vi "LIA Debugging FPGA.vi"() -> ()   [LabVIEW 2017]
uses:
  <instrlib>/_niInstr/Streaming/v1/Common/Stream State.ctl
  <instrlib>/_niInstr/Data Trigger/v1/Shared/Public/Edge Configuration FXP(+-,18,1).ctl
  <instrlib>/_niInstr/Data Trigger/v1/Shared/Public/Edge Configuration Trigger Slope.ctl
  <vilib>/Platform/TimedLoop/XDataNode/timing_clust.ctl
  <vilib>/Platform/TimedLoop/XDataNode/nitl_modes.ctl
  <vilib>/Platform/TimedLoop/XDataNode/wakeup.ctl
  <instrlib>/_niInstr/DSP/v1/Shared/Public/IQ Data.ctl
  <vilib>/rvi/Emulation/niFpgaSctlEmulationGetInTimedLoop.vi
  <vilib>/rvi/Emulation/niFpgaEmulationReportErrorSimple.vi
  <vilib>/rvi/Emulation/niFpgaGetClockAttributes.vi
  <vilib>/rvi/Emulation/niFpgaCriticalErrorInLSC.vi
  <instrlib>/_niInstr/DSP/v1/FPGA/Public/Sub VIs/Frequency Shift/Frequency Shift - 1 spc.vi
  <instrlib>/_niInstr/DSP/v1/FPGA/Public/Sub VIs/Fractional Decimator/Fractional Decimator - 1 spc - 2x oc.vi
  <instrlib>/_niInstr/DSP/v1/FPGA/Public/Sub VIs/Fractional Decimator/Fractional Decimator - 10 cps - 1x oc.vi
  <userlib>/_NI Noise Generation IP/FPGA/Public/Low Level/AWGN FXP23x2.vi
  <instrlib>/_niInstr/DSP/v1/FPGA/Public/Sub VIs/Frequency Shift/Frequency Shift - 2 spc.vi
  <vilib>/rvi/eio/common/nirviEmuTemplateMethod_errors.vi
  <vilib>/Platform/TimedLoop/XDataNode/XDataNode.xnode
  <instrlib>/_niInstr/DSP/v1/Xnodes/Public/Frequency Shift/niInstr DSP v1 Frequency Shift FPGA.xnode
  <vilib>/rvi/FXPMathLib/FxpMul/XNode/nifxpmath_Multiplier.xnode
  <vilib>/rvi/FXPMathLib/FxpAdd/XNode/nifxpmath_Add.xnode
  <vilib>/eio/EIONode/EIONode.xnode
  <vilib>/Platform/TimedLoop/XDataNode/XDNodeRunTimeDep.lvlib
  <instrlib>/_niInstr/Basic Elements/v1/FPGA/niInstr Basic Elements v1 FPGA.lvlib
  <instrlib>/_niInstr/DSP/v1/Shared/niInstr DSP v1 Shared.lvlib
  <instrlib>/_niInstr/DSP/v1/FPGA/niInstr DSP v1 FPGA.lvlib
  Program Files (x86)/National Instruments/LabVIEW 2017/examples/Lock-In Amplifier/_NI PLL IP/FPGA/NI PLL IP FPGA.lvlib
  Program Files (x86)/National Instruments/LabVIEW 2017/examples/Lock-In Amplifier/lib/fpga/Lock-In Amplifier Example FPGA.lvlib
  <instrlib>/_niInstr/Streaming/v1/Common/niInstr Streaming v1 Common.lvlib
  <userlib>/_NI Noise Generation IP/FPGA/NI Noise Generation IP FPGA v2.lvlib
  <vilib>/rvi/FXPMathLib/sim/FxpSim.dll
  <instrlib>/_niInstr/Data Trigger/v1/Shared/niInstr Data Trigger v1 Shared.lvlib
panel:
  in  "lock-in.decimator 1":enum16{"None", "FIR"}(ring)
  in  "lock-in.fir2 fs":fxp<+,48,1>
  in  "nco.enable 0":bool=TRUE
  in  "nco.reset 0":bool
  in  "nco.frequency 0":fxp<+/-,48,0>
  in  "lock-in.fir fs":fxp<+,48,1>
  in  "lock-in.decimator 0":enum16{"None", "CIC", "FIR", "4HB"}(ring)
  in  "dpll.reset 1":bool
  in  "dpll.enable 1":bool
  in  "dpll.q 1":fxp<+/-,48,0>
  in  "dpll.m 1":i8
  in  "dpll.config 1":T1
  out "dpll.vco output 1":fxp<+/-,48,0>
  in  "dpll.channel 1":i32
  in  "dpll.channel 0":i32
  out "dpll.vco output 0":fxp<+/-,48,0>
  in  "dpll.config 0":T1
  in  "dpll.m 0":i8
  in  "dpll.q 0":fxp<+/-,48,0>
  in  "dpll.enable 0":bool
  in  "dpll.reset 0":bool
  in  "lock-in.enable 3":bool
  in  "lock-in.enable 2":bool
  in  "lock-in.enable 1":bool
  in  "lock-in.carrier 3":fxp<+/-,48,0>
  in  "lock-in.carrier 2":fxp<+/-,48,0>
  in  "lock-in.enable 0":bool
  in  "lock-in.channel select 3":i32
  in  "lock-in.carrier select 3":i32
  in  "lock-in.cic config valid 3":bool
  in  "lock-in.cic config 3":cluster{"factor":fxp<+,16,16>, "shift":i16}
  in  "lock-in.reset 3":bool
  out "stream.state 3":T3 caption="stream.state 0"
  out "stream.samples transferred 3":u64 caption="stream.samples transferred 0"
  out "stream.metadata 3":u64 caption="stream.metadata 0"
  in  "stream.num samples 3":u64 caption="stream.num samples 0"
  in  "stream.request state 3":T3 caption="stream.request state 0"
  in  "lock-in.channel select 2":i32
  in  "lock-in.carrier select 2":i32
  in  "lock-in.cic config valid 2":bool
  in  "lock-in.cic config 2":cluster{"factor":fxp<+,16,16>, "shift":i16}
  in  "lock-in.reset 2":bool
  out "stream.state 2":T3 caption="stream.state 0"
  out "stream.samples transferred 2":u64 caption="stream.samples transferred 0"
  out "stream.metadata 2":u64 caption="stream.metadata 0"
  in  "stream.num samples 2":u64 caption="stream.num samples 0"
  in  "stream.request state 2":T3 caption="stream.request state 0"
  out "pll.vco output 0":fxp<+/-,48,0>
  out "pll.vco output 1":fxp<+/-,48,0>
  out "stream.metadata 4":u64 caption="stream.metadata 0"
  out "stream.samples transferred 4":u64 caption="stream.samples transferred 0"
  out "stream.state 4":T3 caption="stream.state 0"
  in  "stream.request state 4":T3 caption="stream.request state 0"
  in  "stream.num samples 4":u64 caption="stream.num samples 0"
  in  "preview.channel select":i32
  in  "ao.reset 3":bool
  in  "ao.carrier 2":fxp<+/-,48,0>=0.010000000000001563
  in  "ao.level 2":fxp<+/-,18,1>
  in  "ao.reset 2":bool
  in  "ao.carrier 1":fxp<+/-,48,0>=0.010000000000001563
  in  "ao.level 1":fxp<+/-,18,1>
  in  "ao.reset 1":bool
  in  "ao.reset 0":bool
  in  "ao.carrier 0":fxp<+/-,48,0>=0.010000000000001563
  in  "ao.level 0":fxp<+/-,18,1>
  in  "lock-in.channel select 1":i32
  in  "lock-in.channel select 0":i32
  in  "stream.request state 1":T3 caption="stream.request state 0"
  in  "stream.num samples 1":u64 caption="stream.num samples 0"
  out "stream.metadata 1":u64 caption="stream.metadata 0"
  out "stream.samples transferred 1":u64 caption="stream.samples transferred 0"
  out "stream.state 1":T3 caption="stream.state 0"
  in  "lock-in.reset 1":bool
  in  "lock-in.cic config 1":cluster{"factor":fxp<+,16,16>, "shift":i16}
  in  "lock-in.cic config valid 1":bool
  in  "lock-in.carrier select 1":i32
  in  "lock-in.carrier select 0":i32
  in  "lock-in.cic config valid 0":bool
  in  "lock-in.cic config 0":cluster{"factor":fxp<+,16,16>, "shift":i16}
  in  "lock-in.reset 0":bool
  in  "lock-in.carrier 1":fxp<+/-,48,0>
  in  "lock-in.carrier 0":fxp<+/-,48,0>
  in  "ao.level 3":fxp<+/-,18,1>
  in  "pll.channel 1":i32
  in  "pll.reset 1":bool
  in  "pll.enable 1":bool
  in  "pll.config 1":T4={"quiescent frequency"=0.10000000000000142, "compensation"=0.0, "psd gain"=-18, "loop filter"={"order"=4, "cutoff"=6}}
  in  "pll.channel 0":i32
  in  "ao.noise gain 3":fxp<+,18,1>=0.01000213623046875
  in  "ao.carrier 3":fxp<+/-,48,0>=0.010000000000001563
  in  "ao.noise seeds 3":fxp<+,23,23>[](array[numeric])=[1.0, 12323.0]
  in  "pll.reset 0":bool
  in  "pll.enable 0":bool
  in  "stream.request state 0":T3
  in  "stream.num samples 0":u64
  out "stream.metadata 0":u64
  out "stream.samples transferred 0":u64
  out "stream.state 0":T3
  in  "pll.config 0":T4={"quiescent frequency"=0.10000000000000142, "compensation"=0.0, "psd gain"=-18, "loop filter"={"order"=4, "cutoff"=6}}
  out "IO Module\\InitDone":bool
  out "IO Module\\User Error":u32
  in  "IO Module\\User Command":u32
  in  "IO Module\\User Command Valid":bool
  out "IO Module\\User Command Ready":bool
  in  "IO Module\\User Command Arg 0":u32
  in  "IO Module\\User Command Arg 1":u32
  out "IO Module\\User Command Error":u16
  out "IO Module\\User Command Return":u32
  out "IO Module\\User Command Return Valid":bool
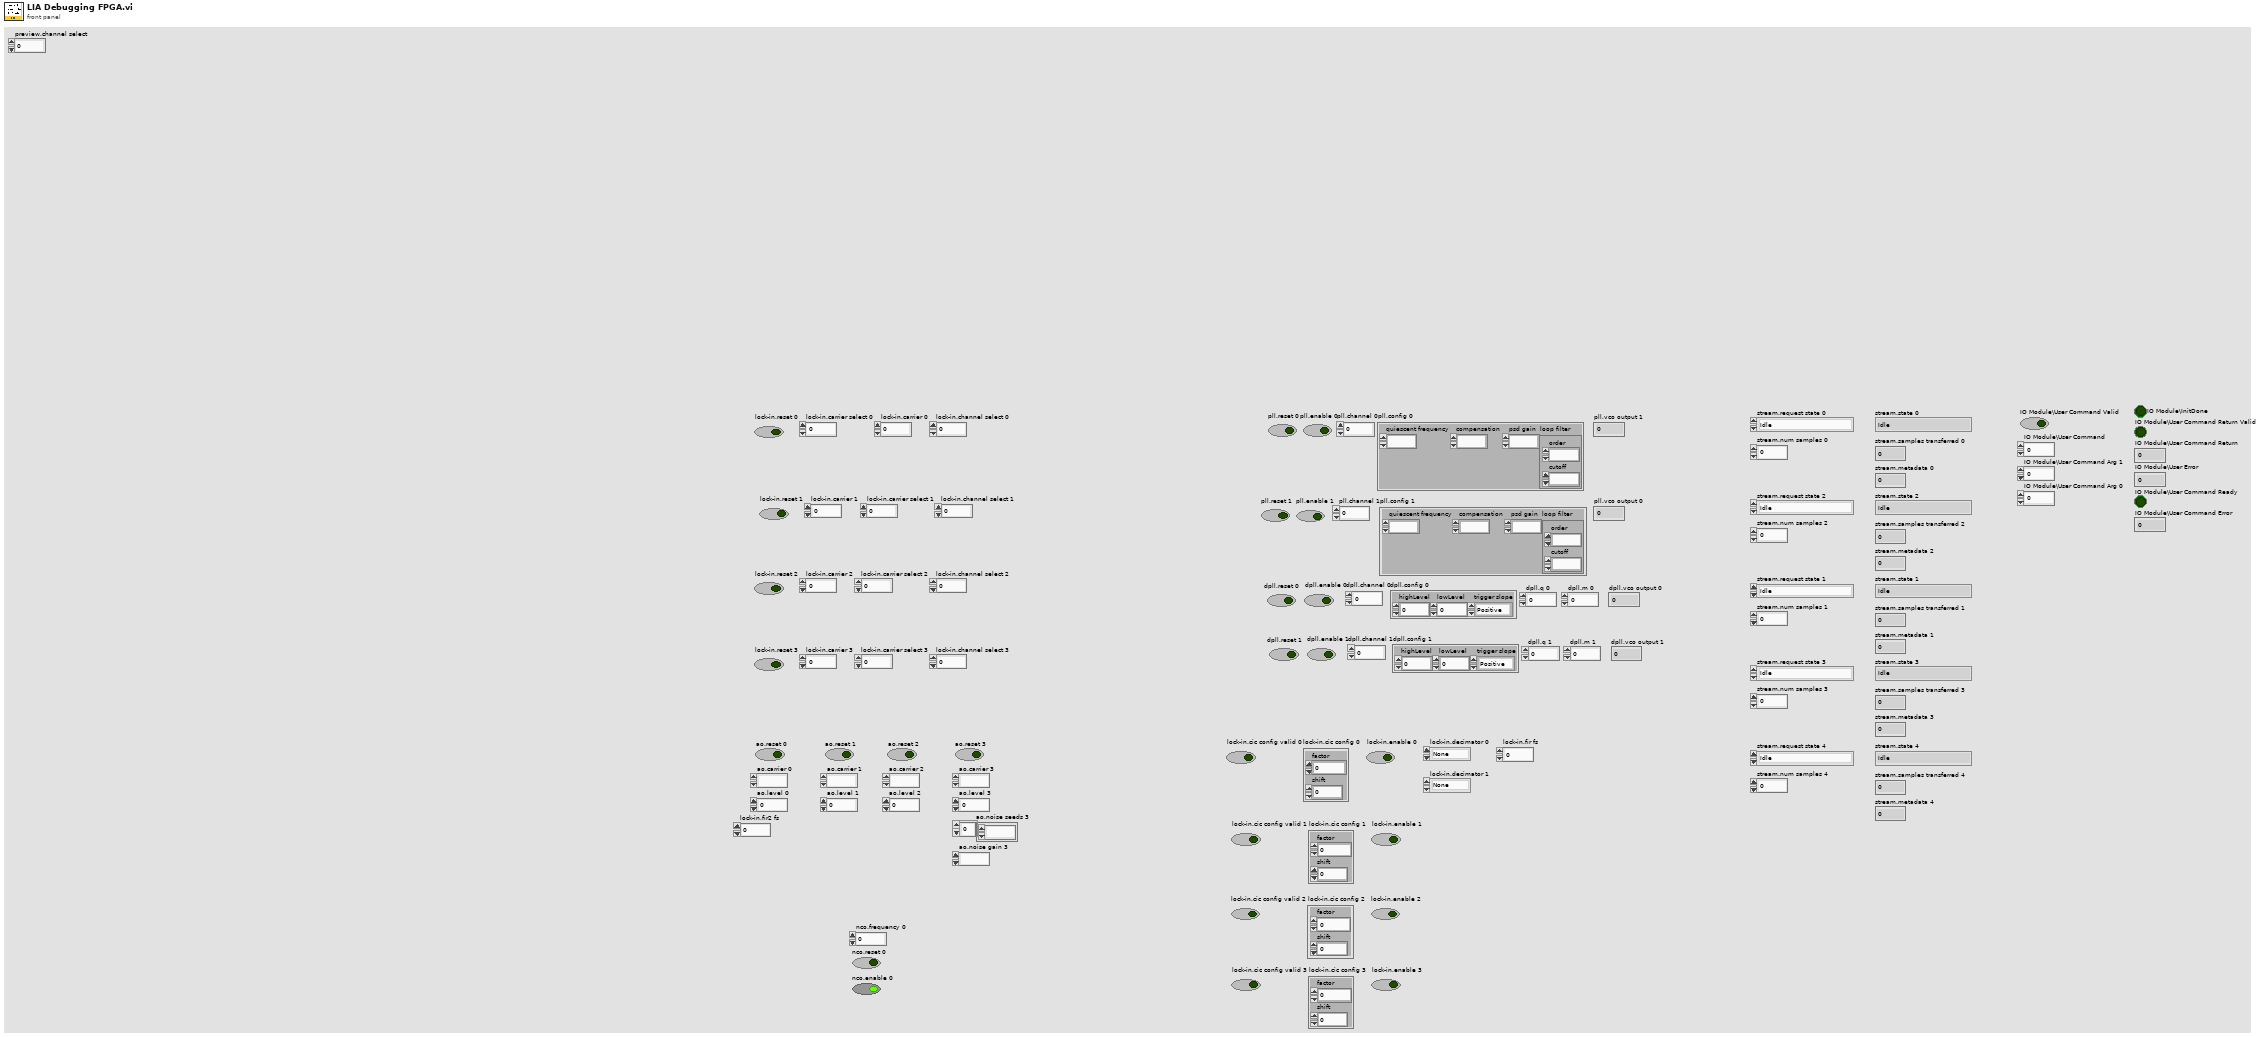
[diagram p1: front panel]
types:
  T1 = typedef "niInstr Data Trigger v1 Shared.lvlib/Edge Configuration FXP(+-,18,1).ctl" = cluster{"highLevel":fxp<+/-,18,1>, "lowLevel":fxp<+/-,18,1>, "trigger slope":T2}
  T2 = typedef "niInstr Data Trigger v1 Shared.lvlib/Edge Configuration Trigger Slope.ctl" = enum8{"Positive", "Negative"}
  T3 = typedef "niInstr Streaming v1 Common.lvlib/Stream State.ctl" = enum8{"Idle", "Finite Transfer", "Continuous", "Done", "Error", "Not Ready", "Cancel"}
  T4 = cluster{"quiescent frequency":fxp<+/-,48,0>, "compensation":fxp<+/-,18,3>, "psd gain":i16, "loop filter":cluster{"order":i32, "cutoff":i8}}
  T5 = typedef "XDNodeRunTimeDep.lvlib/timing_clust.ctl" = cluster{"Expected End [f-1]":u64, "Actual End [f-1]":u64, "Finished Late? [f-1]":bool, "Expected End [i-1]":u64, "Actual End [i-1]":u64, "Finished Late? [i-1]":bool, "Expected Start [i]":u64, "Actual Start [i]":u64, "Expected Start [f]":u64, "Actual Start [f]":u64, "Source Name":string, "Structure Name":string, "Period":i64, "Deadline":i64, "Offset":i64, "Start":i64, "Priority":i32, "Timeout":i32, "Mode":T6, "Wakeup Reason":T7, "Error":errorcluster, "Source Type":string, "Secondary Source Type":string, "Global End Time":u64, "Global Start Time":u64, "Frame Duration":u64, "Iteration Duration":u64, "Assigned CPU":i32, "I/O Scan Engine Mode":u32}
  T6 = typedef "XDNodeRunTimeDep.lvlib/nitl_modes.ctl" = enum32{"No Change", "Process missed periods, maintain original phase", "Discard missed periods, maintain original phase", "Process missed periods, ignore original phase", "Discard missed periods, ignore original phase"}
  T7 = typedef "XDNodeRunTimeDep.lvlib/wakeup.ctl" = enum32{"Normal", "Aborted", "Asynchronous wakeup", "Timing source error", "Timed loop error", "Timeout"}
  T8 = cluster{"stream.num samples 0":u64, "stream.request state 0":T3, "stream.index 0":i16}
  T9 = typedef "niInstr DSP v1 Shared.lvlib/IQ Data.ctl" = cluster{"I":fxp<+/-,18,1>, "Q":fxp<+/-,18,1>, "overflow":bool}
  T10 = cluster{"stream.metadata 0":u64, "stream.samples transferred 0":u64, "stream.state 0":T3}
  T11 = typedef "niInstr DSP v1 Shared.lvlib/IQ Data - 25 bit.ctl" = cluster{"I":fxp<+/-,25,1>, "Q":fxp<+/-,25,1>, "overflow":bool}
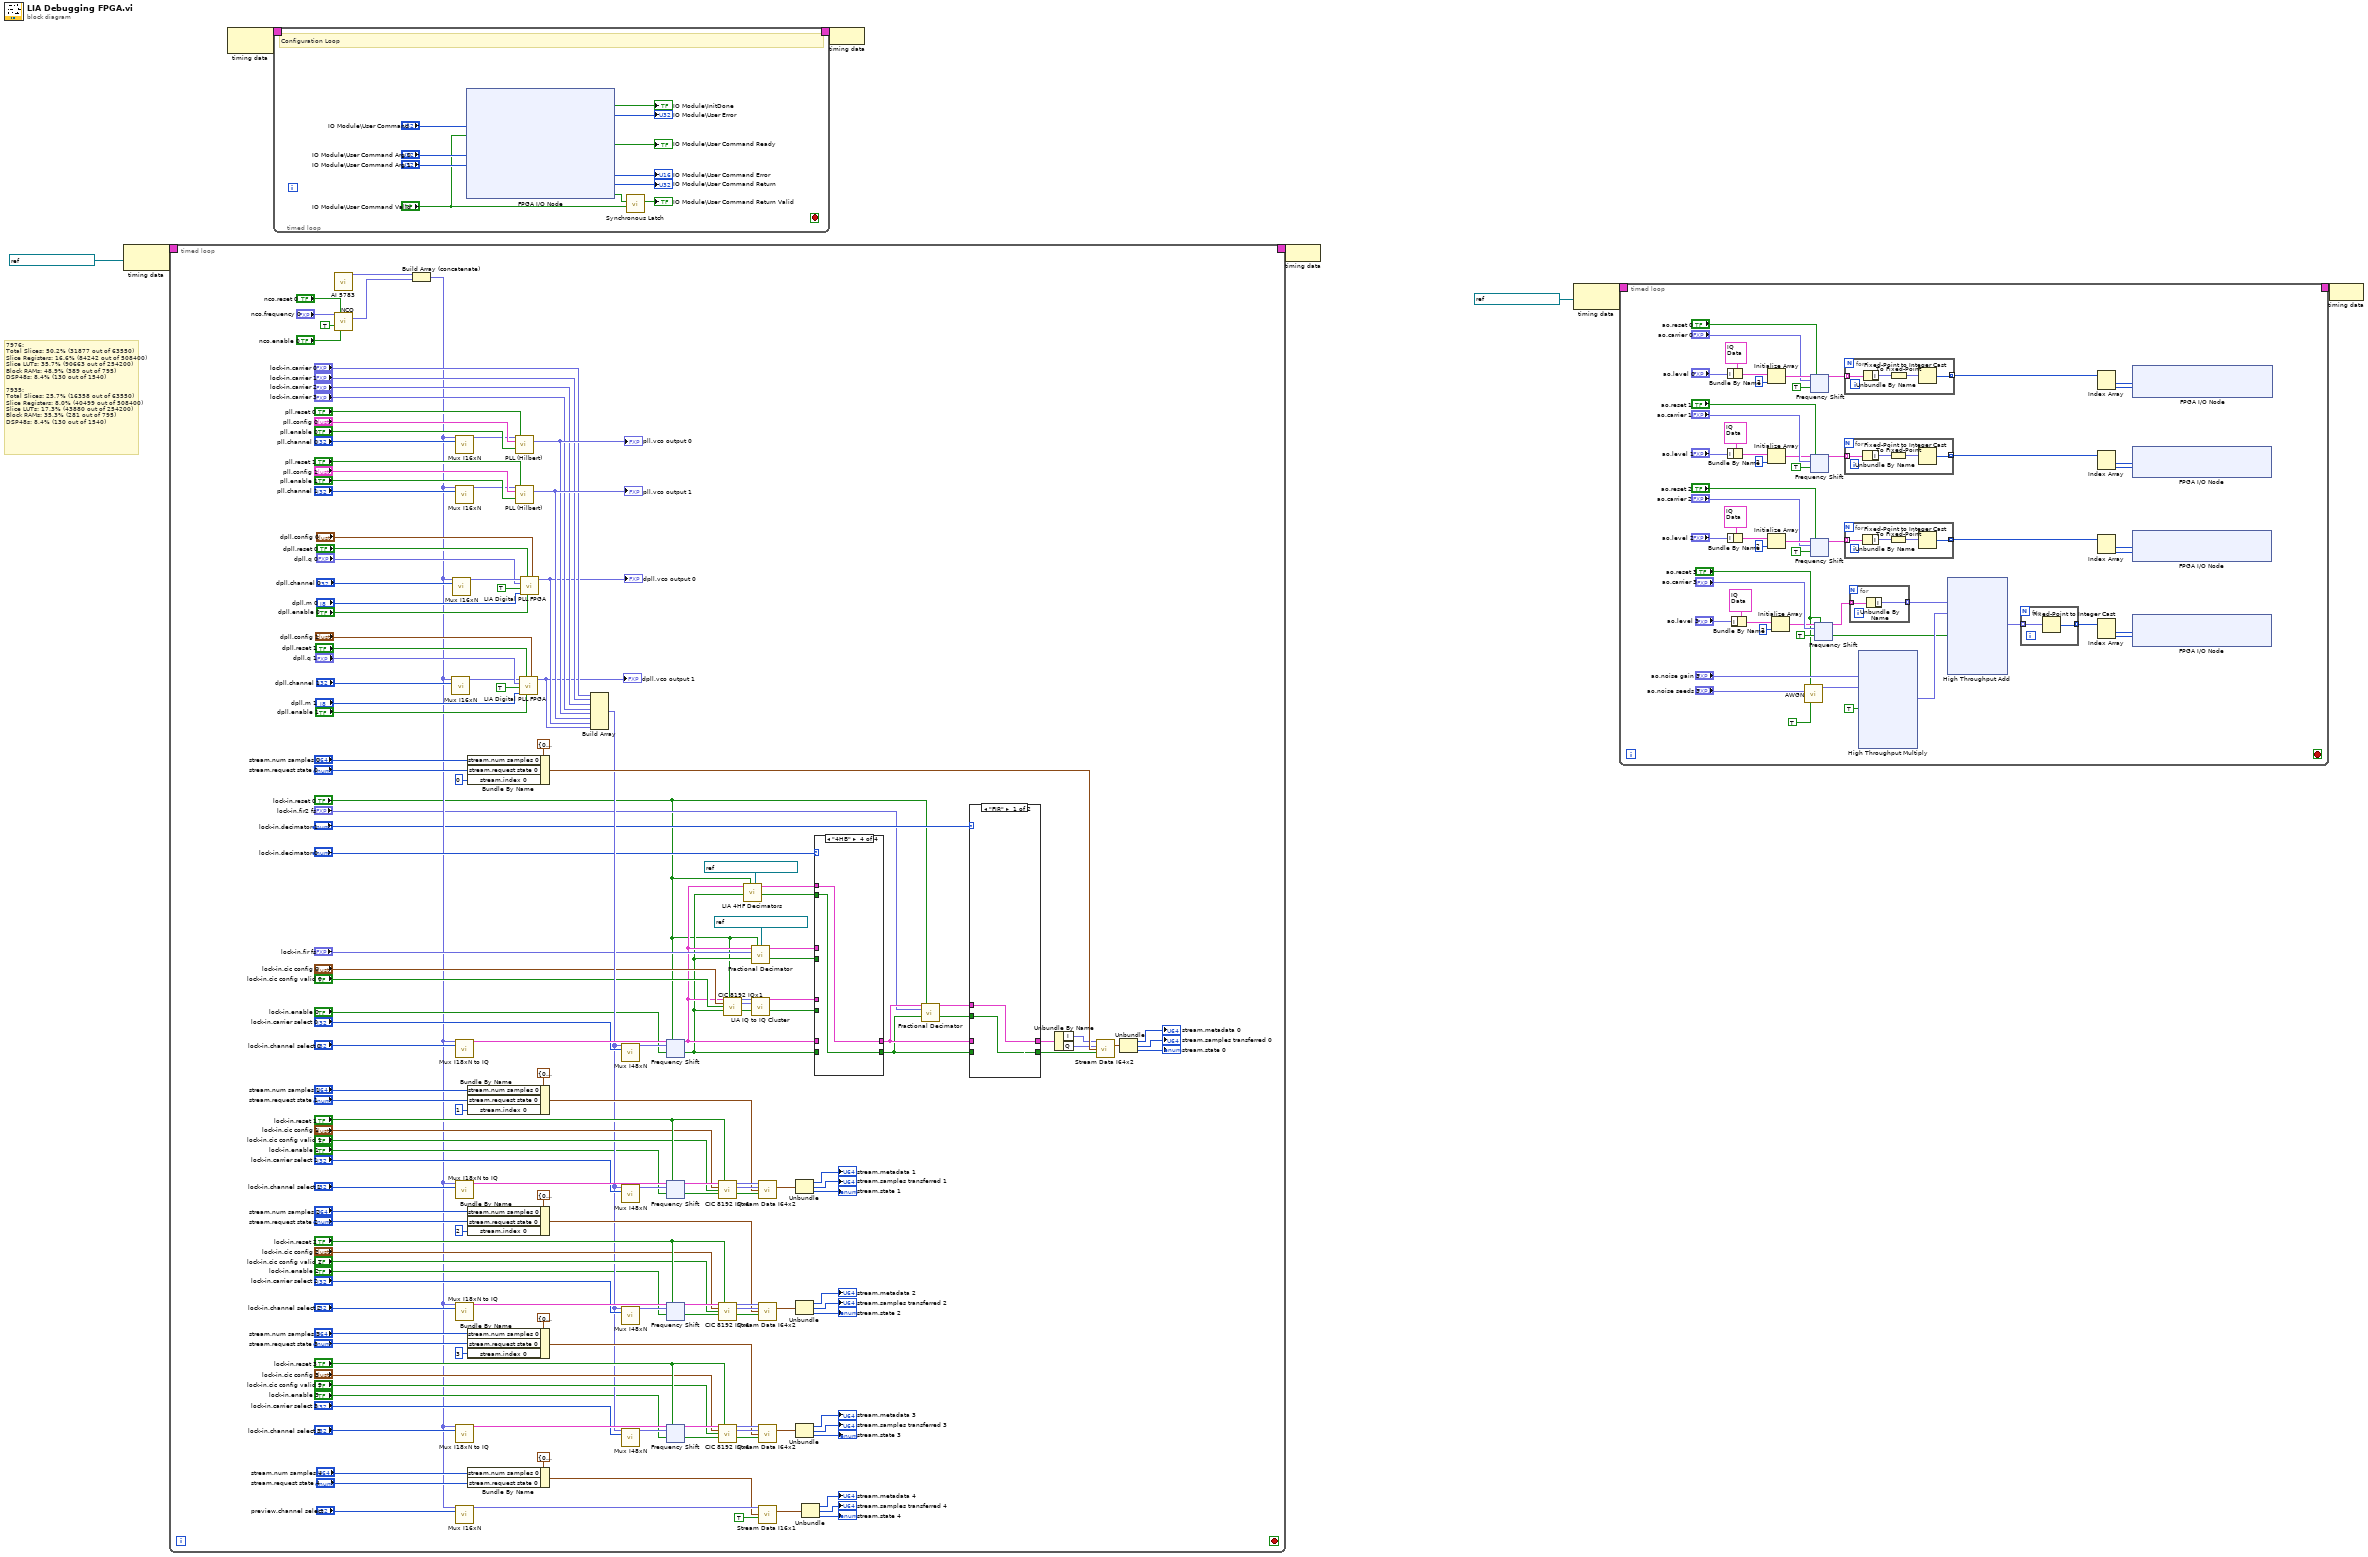
[diagram p0: block diagram]
diagram:
  # "7976:\nTotal Slices: 50.2% (31877 out of 63550)\nSlice Registers: 16.6% (84242 out of 508400)\nSlice LUTs: 35.7% (90663 out of 254200)\nBlock RAMs: 48.9% (389 out of 795)\nDSP48s: 8.4% (130 out of 1540)\n\n7935:\nTotal Slices: 25.7% (16358 out of 63550)\nSlice Registers: 8.0% (40499 out of 508400)\nSlice LUTs: 17.3% (43880 out of 254200)\nBlock RAMs: 35.3% (281 out of 795)\nDSP48s: 8.4% (130 out of 1540)"
  n1 = node-c288(refnum<k21> "IO Module\\Data Clock" ("Source Name")) -> (w8:T5)
  n2 = timed-loop {
    timing: w8 -> [_]
    timing-out: [_] -> w7
    stop <- _ stop-if-true
    n3 = call "AI 5783.vi"() -> ("i18x1"=w43:fxp<+/-,18,1>[])  [unwired: 14 in, 1 out]
    n4 = call <instrlib>:"NCO.vi"("frequency"="nco.frequency 0", "reset"="nco.reset 0", "input valid"=TRUE, "enable (T)"="nco.enable 0") -> ("sine out"=w35:fxp<+/-,18,1>)  [unwired: 9 in, 2 out]
    n5 = Build Array (concatenate)(w43, w35) -> (w36:fxp<+/-,18,1>[])
    n6 = call "Mux I16xN.vi"("i16xn in"=w36, "index"="dpll.channel 1") -> ("i16 out"=w46:fxp<+/-,18,1>)  [unwired: 12 in, 1 out]
    n7 = call "Mux I16xN.vi"("i16xn in"=w36, "index"="dpll.channel 0") -> ("i16 out"=w58:fxp<+/-,18,1>)  [unwired: 12 in, 1 out]
    n8 = call "Mux I16xN.vi"("i16xn in"=w36, "index"="pll.channel 0") -> ("i16 out"=w165:fxp<+/-,18,1>)  [unwired: 12 in, 1 out]
    n9 = call "Mux I16xN.vi"("i16xn in"=w36, "index"="pll.channel 1") -> ("i16 out"=w159:fxp<+/-,18,1>)  [unwired: 12 in, 1 out]
    n10 = call "Mux I18xN to IQ.vi"("i16xn in"=w36, "index"="lock-in.channel select 0") -> ("output"=w158:T9)  [unwired: 12 in, 1 out]
    n11 = call "Mux I18xN to IQ.vi"("i16xn in"=w36, "index"="lock-in.channel select 1") -> ("output"=w145:T9)  [unwired: 12 in, 1 out]
    n12 = call "Mux I18xN to IQ.vi"("i16xn in"=w36, "index"="lock-in.channel select 2") -> ("output"=w111:T9)  [unwired: 12 in, 1 out]
    n13 = call "Mux I18xN to IQ.vi"("i16xn in"=w36, "index"="lock-in.channel select 3") -> ("output"=w90:T9)  [unwired: 12 in, 1 out]
    n14 = call "Mux I16xN.vi"("i16xn in"=w36, "index"="preview.channel select") -> ("i16 out"=w119:fxp<+/-,18,1>)  [unwired: 12 in, 1 out]
    n15 = Bundle By Name(cluster=T8 {"stream.num samples 0"=0, "stream.request state 0"=enum."Idle", "stream.index 0"=0} ("config"), "stream.num samples 0"="stream.num samples 0", "stream.request state 0"="stream.request state 0", "stream.index 0"=i16 0) -> (w148:T8)
    n16 = Bundle By Name(cluster=T8 {"stream.num samples 0"=0, "stream.request state 0"=enum."Idle", "stream.index 0"=0} ("config"), "stream.num samples 0"="stream.num samples 1", "stream.request state 0"="stream.request state 1", "stream.index 0"=i16 1) -> (w127:T8)
    n17 = Bundle By Name(cluster=T8 {"stream.num samples 0"=0, "stream.request state 0"=enum."Idle", "stream.index 0"=0} ("config"), "stream.num samples 0"="stream.num samples 2", "stream.request state 0"="stream.request state 2", "stream.index 0"=i16 2) -> (w93:T8)
    n18 = Bundle By Name(cluster=T8 {"stream.num samples 0"=0, "stream.request state 0"=enum."Idle", "stream.index 0"=0} ("config"), "stream.num samples 0"="stream.num samples 3", "stream.request state 0"="stream.request state 3", "stream.index 0"=i16 3) -> (w72:T8)
    n19 = Bundle By Name(cluster=T8 {"stream.num samples 0"=0, "stream.request state 0"=enum."Idle", "stream.index 0"=0} ("config"), "stream.num samples 0"="stream.num samples 4", "stream.request state 0"="stream.request state 4") -> (w115:T8)
    n20 = call "PLL (Hilbert).vi"("input"=w165, "reset"="pll.reset 0", "config"="pll.config 0", "enable"="pll.enable 0") -> ("output"=w112:fxp<+/-,48,0>)  [unwired: 11 in]
    "pll.vco output 0" <- w112
    n21 = call "PLL (Hilbert).vi"("input"=w159, "reset"="pll.reset 1", "config"="pll.config 1", "enable"="pll.enable 1") -> ("output"=w113:fxp<+/-,48,0>)  [unwired: 11 in]
    "pll.vco output 1" <- w113
    n22 = call "LIA Digital PLL FPGA.vi"("configuration"="dpll.config 1", "arm"="dpll.enable 1", "reset"="dpll.reset 1", "m"="dpll.m 1", "input valid"=TRUE, "q"="dpll.q 1", "I"=w46) -> ("frequency shift"=w42:fxp<+/-,48,0>)  [unwired: 1 in, 3 out]
    "dpll.vco output 1" <- w42
    n23 = call "LIA Digital PLL FPGA.vi"("configuration"="dpll.config 0", "arm"="dpll.enable 0", "reset"="dpll.reset 0", "m"="dpll.m 0", "input valid"=TRUE, "q"="dpll.q 0", "I"=w58) -> ("frequency shift"=w53:fxp<+/-,48,0>)  [unwired: 1 in, 3 out]
    "dpll.vco output 0" <- w53
    n24 = Build Array("lock-in.carrier 0", "lock-in.carrier 1", "lock-in.carrier 2", "lock-in.carrier 3", w112, w113, w53, w42) -> (w69:fxp<+/-,48,0>[])
    n25 = call "Mux I48xN.vi"("i48xn in"=w69, "index"="lock-in.carrier select 0") -> ("i48 out"=w157:fxp<+/-,48,0>)  [unwired: 13 in]
    n26 = call "Mux I48xN.vi"("i48xn in"=w69, "index"="lock-in.carrier select 1") -> ("i48 out"=w144:fxp<+/-,48,0>)  [unwired: 13 in]
    n27 = call "Mux I48xN.vi"("i48xn in"=w69, "index"="lock-in.carrier select 2") -> ("i48 out"=w110:fxp<+/-,48,0>)  [unwired: 13 in]
    n28 = call "Mux I48xN.vi"("i48xn in"=w69, "index"="lock-in.carrier select 3") -> ("i48 out"=w89:fxp<+/-,48,0>)  [unwired: 13 in]
    n29 = xnode "Frequency Shift"("data in"=w158, "reset"="lock-in.reset 0", "frequency shift"=w157, "input valid"="lock-in.enable 0") -> ("data out"=w28:T9, "output valid"=w27:bool)  [unwired: 2 in, 1 out]
    n30 = xnode "Frequency Shift"("data in"=w145, "reset"="lock-in.reset 1", "frequency shift"=w144, "input valid"="lock-in.enable 1") -> ("data out"=w143:T9, "output valid"=w142:bool)  [unwired: 2 in, 1 out]
    n31 = xnode "Frequency Shift"("data in"=w111, "reset"="lock-in.reset 2", "frequency shift"=w110, "input valid"="lock-in.enable 2") -> ("data out"=w109:T9, "output valid"=w108:bool)  [unwired: 2 in, 1 out]
    n32 = xnode "Frequency Shift"("data in"=w90, "reset"="lock-in.reset 3", "frequency shift"=w89, "input valid"="lock-in.enable 3") -> ("data out"=w88:T9, "output valid"=w87:bool)  [unwired: 2 in, 1 out]
    n33 = call "CIC 8192 IQx1.vi"("data"=w143, "reset"="lock-in.reset 1", "config"="lock-in.cic config 1", "config valid"="lock-in.cic config valid 1", "input valid"=w142) -> ("i out"=w138:fxp<+/-,64,1>, "q out"=w137:fxp<+/-,64,1>, "output valid"=w136:bool)  [unwired: 8 in]
    n34 = call "CIC 8192 IQx1.vi"("data"=w109, "reset"="lock-in.reset 2", "config"="lock-in.cic config 2", "config valid"="lock-in.cic config valid 2", "input valid"=w108) -> ("i out"=w104:fxp<+/-,64,1>, "q out"=w103:fxp<+/-,64,1>, "output valid"=w102:bool)  [unwired: 8 in]
    n35 = call "CIC 8192 IQx1.vi"("data"=w88, "reset"="lock-in.reset 3", "config"="lock-in.cic config 3", "config valid"="lock-in.cic config valid 3", "input valid"=w87) -> ("i out"=w83:fxp<+/-,64,1>, "q out"=w82:fxp<+/-,64,1>, "output valid"=w81:bool)  [unwired: 8 in]
    n36 = call "CIC 8192 IQx1.vi"("data"=w28, "reset"="lock-in.reset 0", "config"="lock-in.cic config 0", "config valid"="lock-in.cic config valid 0", "input valid"=w27) -> ("i out"=w17:fxp<+/-,64,1>, "q out"=w16:fxp<+/-,64,1>, "output valid"=w38:bool)  [unwired: 8 in]
    n37 = call "LIA 4HF Decimators.vi"("clock x 2"=refnum<k21> "IO Module\\Data Clock 2x", "reset"="lock-in.reset 0", "input valid"=w27, "data in"=w28) -> ("output valid"=w24:bool, "data out"=w25:T9)  [unwired: 6 in]
    n38 = call "LIA IQ to IQ Cluster.vi"("i in"=w17, "q in"=w16) -> ("data out"=w15:T9)  [unwired: 13 in]
    n39 = call-poly <instrlib>:"Fractional Decimator.vi"("data in"=w28, "reset"="lock-in.reset 0", "clock x 2"=refnum<k21> "IO Module\\Data Clock 2x", "output sample rate"="lock-in.fir fs", "input valid"=w27) -> ("data out"=w29:T9, "output valid"=w30:bool)  [unwired: 8 in, 1 out]
    n40 = call "Stream Data I64x2.vi"("i in"=w138, "q in"=w137, "config"=w127, "input valid"=w136) -> ("status"=w135:T10)  [unwired: 11 in]
    n41 = call "Stream Data I64x2.vi"("i in"=w104, "q in"=w103, "config"=w93, "input valid"=w102) -> ("status"=w101:T10)  [unwired: 11 in]
    n42 = call "Stream Data I64x2.vi"("i in"=w83, "q in"=w82, "config"=w72, "input valid"=w81) -> ("status"=w80:T10)  [unwired: 11 in]
    n43 = call "Stream Data I16x1.vi"("i in"=w119, "config"=w115, "input valid"=TRUE) -> ("status"=w121:T10)  [unwired: 12 in]
    n44 = Unbundle(w135) -> ("stream.metadata 0"=→"stream.metadata 1":u64, "stream.samples transferred 0"=→"stream.samples transferred 1":u64, "stream.state 0"=→"stream.state 1":T3)
    n45 = Unbundle(w101) -> ("stream.metadata 0"=→"stream.metadata 2":u64, "stream.samples transferred 0"=→"stream.samples transferred 2":u64, "stream.state 0"=→"stream.state 2":T3)
    n46 = Unbundle(w80) -> ("stream.metadata 0"=→"stream.metadata 3":u64, "stream.samples transferred 0"=→"stream.samples transferred 3":u64, "stream.state 0"=→"stream.state 3":T3)
    n47 = Unbundle(w121) -> ("stream.metadata 0"=→"stream.metadata 4":u64, "stream.samples transferred 0"=→"stream.samples transferred 4":u64, "stream.state 0"=→"stream.state 4":T3)
    n48 = case shown="\"4HB\"" "lock-in.decimator 0" {
      tunnel: [w174 w176 w178 w180] -> w11
      tunnel: w38 -> [_ w176 _ _]
      tunnel: w30 -> [_ _ w178 _]
      tunnel: w27 -> [w174 _ _ _]
      tunnel: w29 -> [_ _ w177 _]
      tunnel: w28 -> [w173 _ _ _]
      tunnel: w25 -> [_ _ _ w179]
      tunnel: w24 -> [_ _ _ w180]
      tunnel: [w173 w175 w177 w179] -> w14
      tunnel: w15 -> [_ w175 _ _]
      frame "None", Default {
      }
      frame "CIC" {
      }
      frame "FIR" {
      }
      frame "4HB" {
      }
    }
    n49 = call-poly <instrlib>:"Fractional Decimator.vi"("data in"=w14, "reset"="lock-in.reset 0", "output sample rate"="lock-in.fir2 fs", "input valid"=w11) -> ("data out"=w13:T11, "output valid"=w12:bool)  [unwired: 9 in, 1 out]
    n50 = case shown="\"FIR\"" "lock-in.decimator 1" {
      tunnel: [w169 w172] -> w23
      tunnel: w11 -> [_ w172]
      tunnel: w14 -> [_ w171]
      tunnel: [w170 w171] -> w21
      tunnel: w13 -> [w170 _]
      tunnel: w12 -> [w169 _]
      frame "FIR" {
      }
      frame "None", Default {
      }
    }
    n51 = Unbundle By Name(w21) -> ("I"=w20:fxp<+/-,25,1>, "Q"=w19:fxp<+/-,25,1>)
    n52 = call "Stream Data I64x2.vi"("i in"=w20, "q in"=w19, "config"=w148, "input valid"=w23) -> ("status"=w156:T10)  [unwired: 11 in]
    n53 = Unbundle(w156) -> ("stream.metadata 0"=→"stream.metadata 0":u64, "stream.samples transferred 0"=→"stream.samples transferred 0":u64, "stream.state 0"=→"stream.state 0":T3)
  }
  n54 = node-c288() -> (w2:T5)  [unwired: 1 in]
  n55 = timed-loop {
    timing: w2 -> [_]
    timing-out: [_] -> w1
    stop <- _ stop-if-true
    # "Configuration Loop"
    n56 = xnode "FPGA I/O Node"("IO Module\\User Command"="IO Module\\User Command", "IO Module\\User Command Valid"="IO Module\\User Command Valid", "IO Module\\User Command Arg 0"="IO Module\\User Command Arg 0", "IO Module\\User Command Arg 1"="IO Module\\User Command Arg 1") -> ("IO Module\\InitDone"=→"IO Module\\InitDone":bool, "IO Module\\Clip Error Code"=→"IO Module\\User Error":u32, "IO Module\\User Command Ready"=→"IO Module\\User Command Ready":bool, "IO Module\\User Command Error"=→"IO Module\\User Command Error":u16, "IO Module\\User Command Return"=→"IO Module\\User Command Return":u32, "IO Module\\User Command Return Valid"=w220:bool)  [unwired: 10 in, 10 out]
    n57 = call <instrlib>:"Synchronous Latch.vi"("clear"="IO Module\\User Command Valid", "set"=w220) -> ("out"=→"IO Module\\User Command Return Valid":bool)  [unwired: 9 in]
  }
  n58 = node-c288(w1) -> ()
  n59 = node-c288(w7) -> ()
  n60 = node-c288(refnum<k21> "IO Module\\Data Clock" ("Source Name")) -> (w5:T5)
  n61 = timed-loop {
    timing: w5 -> [_]
    timing-out: [_] -> w4
    stop <- _ stop-if-true
    n62 = Bundle By Name(cluster=T9 {"I"=0.0, "Q"=0.0, "overflow"=FALSE} ("output"), "I"="ao.level 1") -> (w253:T9)
    n63 = Bundle By Name(cluster=T9 {"I"=0.0, "Q"=0.0, "overflow"=FALSE} ("output"), "I"="ao.level 2") -> (w243:T9)
    n64 = Bundle By Name(cluster=T9 {"I"=0.0, "Q"=0.0, "overflow"=FALSE} ("output"), "I"="ao.level 0") -> (w268:T9)
    n65 = Bundle By Name(cluster=T9 {"I"=0.0, "Q"=0.0, "overflow"=FALSE} ("output"), "I"="ao.level 3") -> (w277:T9)
    n66 = Initialize Array(w253, 2 ("dimension size")) -> (w249:T9[])
    n67 = Initialize Array(w243, 2 ("dimension size")) -> (w247:T9[])
    n68 = Initialize Array(w268, 2 ("dimension size")) -> (w272:T9[])
    n69 = Initialize Array(w277, 2 ("dimension size")) -> (w273:T9[])
    n70 = call-poly <userlib>:"AWGN.vi"("reset"="ao.reset 3", "seeds"="ao.noise seeds 3", "ready"=TRUE) -> ("output 0"=w280:fxp<+/-,23,4>[])  [unwired: 10 in, 2 out]
    n71 = xnode "Frequency Shift"("data in"=w249, "reset"="ao.reset 1", "frequency shift"="ao.carrier 1", "input valid"=TRUE) -> ("data out"=w257:T9[])  [unwired: 2 in, 2 out]
    n72 = xnode "Frequency Shift"("data in"=w247, "reset"="ao.reset 2", "frequency shift"="ao.carrier 2", "input valid"=TRUE) -> ("data out"=w239:T9[])  [unwired: 2 in, 2 out]
    n73 = xnode "Frequency Shift"("data in"=w272, "reset"="ao.reset 0", "frequency shift"="ao.carrier 0", "input valid"=TRUE) -> ("data out"=w264:T9[])  [unwired: 2 in, 2 out]
    n74 = xnode "Frequency Shift"("data in"=w273, "reset"="ao.reset 3", "frequency shift"="ao.carrier 3", "input valid"=TRUE) -> ("data out"=w288:T9[], "output valid"=w285:bool)  [unwired: 2 in, 1 out]
    n75 = for {
      tunnel: w257 -> [w304] mode=indexing
      tunnel: [w305] -> w258 mode=indexing
      n76 = Unbundle By Name(w304) -> ("I"=w303:fxp<+/-,18,1>)
      n77 = To Fixed-Point(number=w303) -> (fixed-point=w302:fxp<+/-,16,1>)  [unwired: 1 in]
      n78 = Fixed-Point to Integer Cast(1:w302) -> (0:w305:i16)
    }
    n79 = for {
      tunnel: w239 -> [w291] mode=indexing
      tunnel: [w292] -> w238 mode=indexing
      n80 = Unbundle By Name(w291) -> ("I"=w290:fxp<+/-,18,1>)
      n81 = To Fixed-Point(number=w290) -> (fixed-point=w289:fxp<+/-,16,1>)  [unwired: 1 in]
      n82 = Fixed-Point to Integer Cast(1:w289) -> (0:w292:i16)
    }
    n83 = for {
      tunnel: w264 -> [w317] mode=indexing
      tunnel: [w318] -> w263 mode=indexing
      n84 = Unbundle By Name(w317) -> ("I"=w316:fxp<+/-,18,1>)
      n85 = To Fixed-Point(number=w316) -> (fixed-point=w315:fxp<+/-,16,1>)  [unwired: 1 in]
      n86 = Fixed-Point to Integer Cast(1:w315) -> (0:w318:i16)
    }
    n87 = for {
      tunnel: w288 -> [w331] mode=indexing
      tunnel: [w330] -> w284 mode=indexing
      n88 = Unbundle By Name(w331) -> ("I"=w330:fxp<+/-,18,1>)
    }
    n89 = xnode ("High Throughput Multiply")("x"="ao.noise gain 3", "y"=w280, "input valid"=TRUE) -> ("x*y"=w287:fxp<+/-,41,5>[])  [unwired: 1 in, 2 out]
    n90 = xnode ("High Throughput Add")("x"=w284, "y"=w287, "input valid"=w285) -> ("x+y"=w279:fxp<+/-,16,1>[])  [unwired: 1 in, 2 out]
    n91 = for {
      tunnel: w279 -> [w329] mode=indexing
      tunnel: [w328] -> w248 mode=indexing
      n92 = Fixed-Point to Integer Cast(1:w329) -> (0:w328:i16)
    }
    n93 = Index Array(array=w263) -> (element #1=w262:i16, element #2=w261:i16)  [unwired: 2 in]
    n94 = Index Array(array=w258) -> (element #1=w259:i16, element #2=w260:i16)  [unwired: 2 in]
    n95 = Index Array(array=w238) -> (element #1=w237:i16, element #2=w236:i16)  [unwired: 2 in]
    n96 = Index Array(array=w248) -> (element #1=w235:i16, element #2=w234:i16)  [unwired: 2 in]
    n97 = xnode "FPGA I/O Node"("IO Module\\AO 1 Data N-1 Data Clock"=w259, "IO Module\\AO 1 Data N Data Clock"=w260) -> ()  [unwired: 2 in, 2 out]
    n98 = xnode "FPGA I/O Node"("IO Module\\AO 2 Data N-1 Data Clock"=w237, "IO Module\\AO 2 Data N Data Clock"=w236) -> ()  [unwired: 2 in, 2 out]
    n99 = xnode "FPGA I/O Node"("IO Module\\AO 3 Data N-1 Data Clock"=w235, "IO Module\\AO 3 Data N Data Clock"=w234) -> ()  [unwired: 2 in, 2 out]
    n100 = xnode "FPGA I/O Node"("IO Module\\AO 0 Data N-1 Data Clock"=w262, "IO Module\\AO 0 Data N Data Clock"=w261) -> ()  [unwired: 2 in, 2 out]
  }
  n101 = node-c288(w4) -> ()
